vi "EVT HLP Get U Char By Pointer.vi"(11 "ptr":i64) -> (3 "function return":u8)   [LabVIEW 2019, in "EmergentCameraC.lvlib"]
doc: "EMERGENTCAMERAC_API unsigned char EVT_HLP_GetUCharByPointer(UCHAR_PTR ptr);"
uses:
  EmergentCameraC.lvlib
  emergentInstall_Windows/win64/eSDK/bin/EmergentCameraC.dll
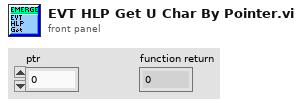
[diagram p1: front panel]
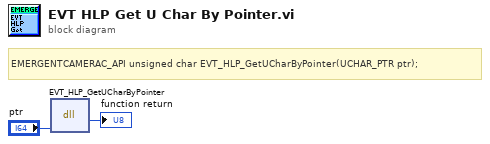
[diagram p0: block diagram]
diagram:
  # "EMERGENTCAMERAC_API unsigned char EVT_HLP_GetUCharByPointer(UCHAR_PTR ptr);"
  n1 = dll-call lib="E:/emergent/host-new_QT/emergentInstall_Windows/win64/eSDK/bin/EmergentCameraC.*" fn="EVT_HLP_GetUCharByPointer"("ptr"="ptr") -> (→"function return":u8)  [unwired: 4 in, 2 out]
